vi "ZonalValues.vi"(8 "error in (no error)":errorcluster, 10 "HasoSlopes In":refnum<class "HasoSlopes.lvclass">, 11 "HASO4_3 in":refnum<class "HASO4_3.lvclass">) -> (0 "error out":errorcluster, 1 "Phase values 2":sgl[][](graph), 2 "HasoSlopesOut":refnum<class "HasoSlopes.lvclass">, 3 "HASO4_3 out":refnum<class "HASO4_3.lvclass">, 4 "Pamameter":T1, 6 "StatisticsData":T2)   [LabVIEW 2020, in "HASO4_3.lvclass"]
uses:
  HASO4_3.lvclass
  WaveKit/Classes/HasoSlopes/HasoSlopes.lvclass
  WaveKit/Controls/StatisticsData.ctl
  WaveKit/Classes/Pupil/Pupil.lvclass
  WaveKit/Classes/Phase/Phase.lvclass
  WaveKit/Classes/HasoData/HasoData.lvclass
  WaveKit/Classes/ComputePhaseSet/ComputePhaseSet.lvclass
  WaveKit/Controls/Point2Df.ctl
  WaveKit/Controls/WavefrontReconstructionMode.ctl
  HASO4_3.lvclass/HASO4_3.ctl
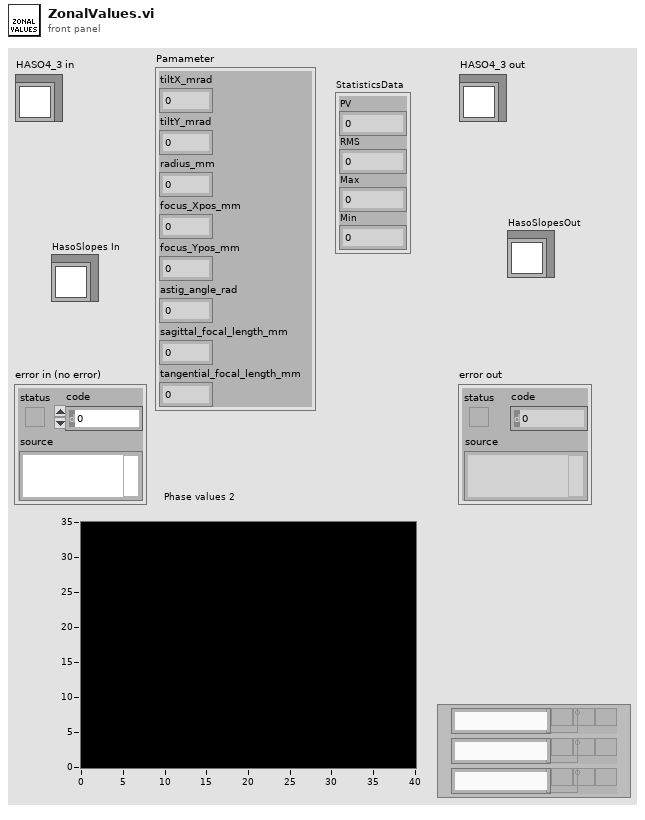
[diagram p1: front panel]
types:
  T1 = cluster{"tiltX_mrad":sgl, "tiltY_mrad":dbl, "radius_mm":sgl, "focus_Xpos_mm":sgl, "focus_Ypos_mm":sgl, "astig_angle_rad":sgl, "sagittal_focal_length_mm":sgl, "tangential_focal_length_mm":sgl}
  T2 = typedef "StatisticsData.ctl" = cluster{"PV":sgl, "RMS":dbl, "Max":sgl, "Min":sgl}
  T3 = typedef "WavefrontReconstructionMode.ctl" = enum16{"None", "Modal_Legendre", "Modal_Zernike", "Zonal", "Modal_Zonal_Zernike", "Modal_Zonal_Legendre"}
  T4 = typedef "Point2Df.ctl" = cluster{"X":sgl, "Y":sgl}
  T5 = typedef "Point2D.ctl" = cluster{"X":u32, "Y":u32}
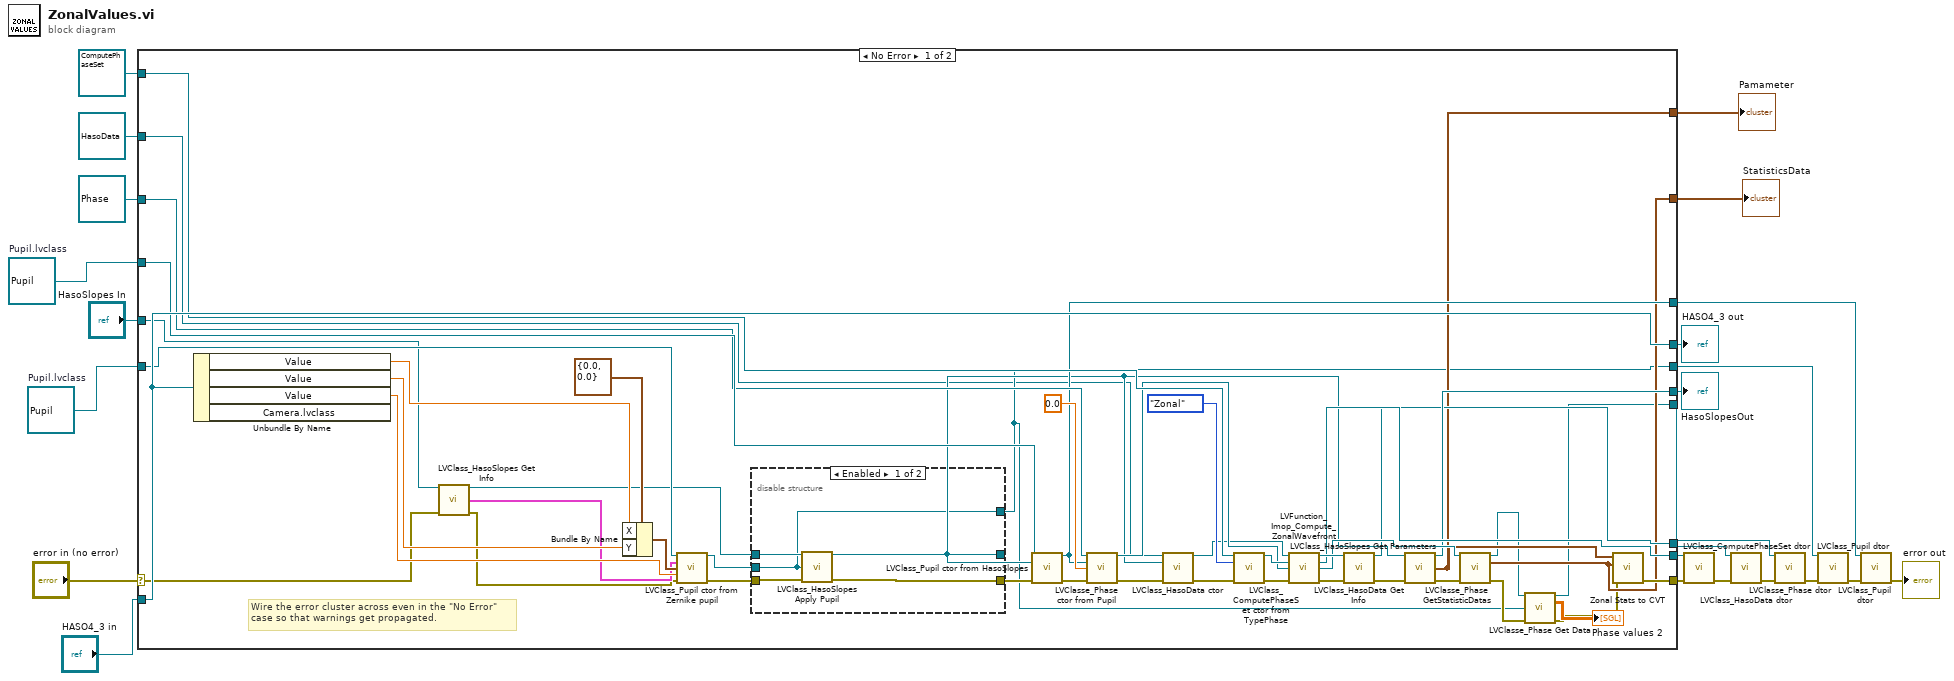
[diagram p0: block diagram]
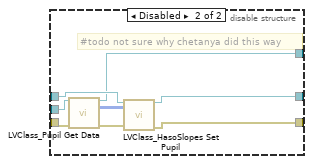
[diagram p2: hidden frame]
diagram:
  w18 = refnum<class "Pupil.lvclass"> refnum  # Pupil.lvclass
  w19 = refnum<class "Pupil.lvclass"> refnum  # Pupil.lvclass
  n1 = case shown="No Error" "error in (no error)" {
    selector: "error in (no error)" -> [w25 w91]
    tunnel: [w42 w91] -> w10
    tunnel: [w70 w90] -> w21
    tunnel: "HASO4_3 in" -> [w70 w90]
    tunnel: "HasoSlopes In" -> [w28 w88]
    tunnel: w19 -> [w66 w89]
    tunnel: w18 -> [w62 w84]
    tunnel: refnum<class "Phase.lvclass"> refnum ("Phase.lvclass") -> [w61 w86]
    tunnel: refnum<class "HasoData.lvclass"> refnum ("HasoData.lvclass") -> [w29 w85]
    tunnel: refnum<class "ComputePhaseSet.lvclass"> refnum ("ComputePhaseSet.lvclass") -> [w56 w87]
    tunnel: [w48 w87] -> w14
    tunnel: [w47 w88] -> w4
    tunnel: [w30 w89] -> w13
    tunnel: [w45 w84] -> w12
    tunnel: [w34 w86] -> w8
    tunnel: [w43 w85] -> w11
    tunnel: [w37 _] -> w2
    tunnel: [w36 _] -> w1
    frame No Error {
      # "Wire the error cluster across even in the \"No Error\"\ncase so that warnings get propagated."
      n2 = Unbundle By Name(w70) -> ("Value"=w68:dbl, "Value"=w67:dbl, "Value"=w64:dbl)  [unwired: 1 out]
      n3 = call "LVClass_HasoSlopes Get Info.vi"("HasoSlopes in"=w28, "error in (no error)"=w25) -> ("HasoSlopes out"=w26:refnum<class "HasoSlopes.lvclass">, "dimension"=w27:cluster{"size":T5, "step":T4}, "error out"=w24:errorcluster)  [unwired: 9 in, 2 out]
      n4 = Bundle By Name(cluster=T4 {"X"=0.0, "Y"=0.0} ("Pupil Dims.center"), "X"=w68, "Y"=w67) -> (w65:T4)
      n5 = call "LVClass_Pupil ctor from Zernike pupil.vi"("Pupil (const)"=w66, "Dimensions_um"=w27, "center"=w65, "rayon"=w64, "error constant"=w24) -> ("Pupil (new)"=w46:refnum<class "Pupil.lvclass">, "error IO"=w63:errorcluster)  [unwired: 9 in]
      n6 = disable-structure shown="Enabled" {
        disable-tunnel: w26 -> [w75 w80]
        disable-tunnel: w63 -> [w74 w82]
        disable-tunnel: [w73 w78] -> w59
        disable-tunnel: w46 -> [w71 w83]
        disable-tunnel: [w72 w77] -> w39
        disable-tunnel: [w71 w76] -> w30
        frame Enabled {
          n7 = call "LVClass_HasoSlopes Apply Pupil.vi"("HasoSlopes in"=w75, "Pupil IN"=w71, "error in (no error)"=w74) -> ("HasoSlopes out"=w72:refnum<class "HasoSlopes.lvclass">, "error out"=w73:errorcluster)  [unwired: 11 in]
        }
        frame Disabled {
          # "#todo not sure why chetanya did this way"
          n8 = call "LVClass_Pupil Get Data.vi"("Pupil in"=w83, "error in (no error)"=w82) -> ("Pupil out"=w76:refnum<class "Pupil.lvclass">, "Data"=w81:i32[][], "error out"=w79:errorcluster)  [unwired: 11 in]
          n9 = call "LVClass_HasoSlopes Set Pupil.vi"("HasoSlopes in"=w80, "Pupil"=w81, "error in (no error)"=w79) -> ("HasoSlopes out"=w77:refnum<class "HasoSlopes.lvclass">, "error out"=w78:errorcluster)  [unwired: 11 in]
        }
      }
      n10 = call "LVClass_Pupil ctor from HasoSlopes.vi"("Pupil (const)"=w62, "HasoSlopes"=w39, "error in (no error)"=w59) -> ("Pupil (new)"=w45:refnum<class "Pupil.lvclass">, "error out"=w58:errorcluster)  [unwired: 10 in, 1 out]
      n11 = call "LVClasse_Phase ctor from Pupil.vi"("Phase (const)"=w61, "Pupil"=w45, "coef"=sgl 0.0, "error in (no error)"=w58) -> ("Phase (new)"=w54:refnum<class "Phase.lvclass">, "error out"=w41:errorcluster)  [unwired: 9 in, 1 out]
      n12 = call "LVClass_HasoData ctor.vi"("HasoData (const)"=w29, "HasoSlopes"=w39, "error in (no error)"=w41) -> ("HasoData (new)"=w38:refnum<class "HasoData.lvclass">, "error out"=w40:errorcluster)  [unwired: 10 in, 1 out]
      n13 = call "LVClass_ComputePhaseSet ctor from TypePhase.vi"("ComputePhaseSet (const)"=w56, "TypePhase"=WavefrontReconstructionMode."Zonal", "error in (no error)"=w40) -> ("ComputePhaseSet (new)"=w55:refnum<class "ComputePhaseSet.lvclass">, "error out"=w53:errorcluster)  [unwired: 11 in]
      n14 = call "LVFunction_Imop_Compute_ZonalWavefront.vi"("HasoData.lvclass"=w38, "ComputePhaseSet.lvclass"=w55, "Phase"=w54, "error constant"=w53) -> ("HasoData.lvclass (dup)"=w51:refnum<class "HasoData.lvclass">, "ComputePhaseSet.lvclass 2"=w48:refnum<class "ComputePhaseSet.lvclass">, "Phase"=w49:refnum<class "Phase.lvclass">, "error out"=w52:errorcluster)  [unwired: 8 in]
      n15 = call "LVClass_HasoData Get Info.vi"("HasoData in"=w51, "error in (no error)"=w52) -> ("HasoData out"=w43:refnum<class "HasoData.lvclass">, "error out"=w50:errorcluster)  [unwired: 11 in, 1 out]
      n16 = call "LVClass_HasoSlopes Get Parameters.vi"("HasoSlopes in"=w39, "error in (no error)"=w50) -> ("HasoSlopes out"=w47:refnum<class "HasoSlopes.lvclass">, "Pamameter"=w37:T1, "error out"=w44:errorcluster)  [unwired: 11 in]
      n17 = call "LVClasse_Phase GetStatisticDatas.vi"("Phase in"=w49, "error in (no error)"=w44) -> ("Phase out"=w35:refnum<class "Phase.lvclass">, "StatisticsData"=w36:T2, "error out"=w32:errorcluster)  [unwired: 11 in]
      n18 = call "LVClasse_Phase Get Data.vi"("Phase in"=w35, "Pupil"=w30, "error in (no error)"=w32) -> ("Phase out"=w34:refnum<class "Phase.lvclass">, "data"=→"Phase values 2":sgl[][], "error out"=w31:errorcluster)  [unwired: 9 in, 1 out]
      n19 = call "Zonal Stats to CVT.vi"("error in (no error)"=w31, "StatisticsData"=w36, "Pamameter"=w37) -> ("error out"=w42:errorcluster)  [unwired: 8 in]
    }
    frame Error {
    }
  }
  "HASO4_3 out" <- w21
  "HasoSlopesOut" <- w4
  "Pamameter" <- w2
  "StatisticsData" <- w1
  n20 = call "LVClass_ComputePhaseSet dtor.vi"("ComputePhaseSet in"=w14, "error in (no error)"=w10) -> ("error out"=w9:errorcluster)  [unwired: 12 in, 1 out]
  n21 = call "LVClass_HasoData dtor.vi"("HasoData in"=w11, "error in (no error)"=w9) -> ("error out"=w3:errorcluster)  [unwired: 12 in, 1 out]
  n22 = call "LVClasse_Phase dtor.vi"("Phase in"=w8, "error in (no error)"=w3) -> ("error out"=w7:errorcluster)  [unwired: 12 in, 1 out]
  n23 = call "LVClass_Pupil dtor.vi"("Pupil in"=w13, "error in (no error)"=w7) -> ("error out"=w6:errorcluster)  [unwired: 12 in, 1 out]
  n24 = call "LVClass_Pupil dtor.vi"("Pupil in"=w12, "error in (no error)"=w6) -> ("error out"=→"error out":errorcluster)  [unwired: 12 in, 1 out]
